vi "Weather Underground - Get Current Temperature.vi"(8 "Error In":errorcluster, 10 "Zip Code":string, 11 "API Key":string) -> (0 "Error Out":errorcluster, 2 "Temperature (F)":i32)   [LabVIEW 2014]
uses:
  <vilib>/httpClient/LabVIEWHTTPClient.lvlib
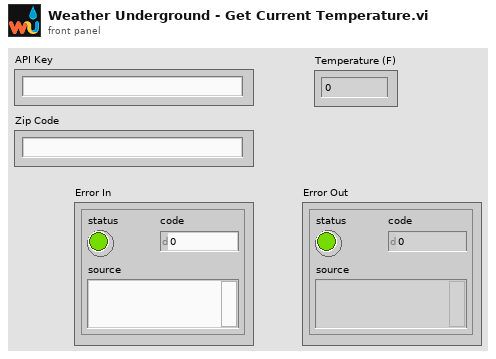
[diagram p1: front panel]
types:
  T1 = cluster{"current_observation":cluster{"temp_f":i32}}
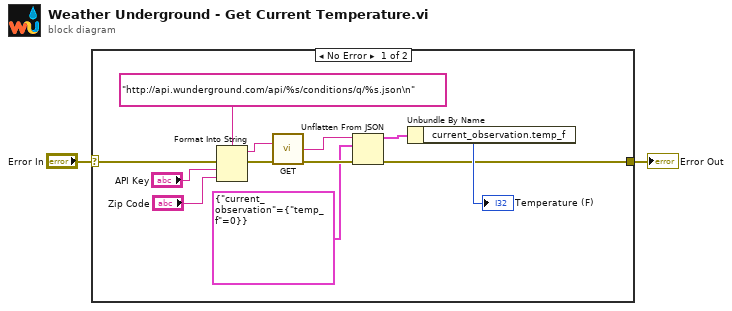
[diagram p0: block diagram]
diagram:
  n1 = case shown="No Error" "Error In" {
    selector: "Error In" -> [w13 w15]
    tunnel: [w3 w15] -> w1
    frame No Error {
      n2 = Format Into String(format string="http://api.wunderground.com/api/%s/conditions/q/%s.json\n", error in=w13, "API Key", "Zip Code") -> (resulting string=w10:string, error out=w9:errorcluster)  [unwired: 1 in]
      n3 = call <vilib>:"GET.vi"("url"=w10, "error in (no error)"=w9) -> ("body"=w7:string, "error out"=w8:errorcluster)  [unwired: 10 in, 2 out]
      n4 = Unflatten From JSON(JSON string=w7, type and defaults=T1 {"current_observation"={"temp_f"=0}}, error in (no error)=w8) -> (value=w5:T1, error out=w3:errorcluster)  [unwired: 4 in]
      n5 = Unbundle By Name(w5) -> ("current_observation.temp_f"=→"Temperature (F)":i32)
    }
    frame Error {
    }
  }
  "Error Out" <- w1
